vi "popElement.vi"(10 "result string 3":string, 11 "type in":i32) -> (1 "element":string, 2 "rest":string, 3 "type out":i32)   [LabVIEW 2023]
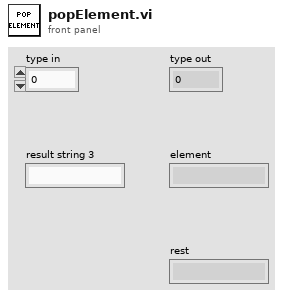
[diagram p1: front panel]
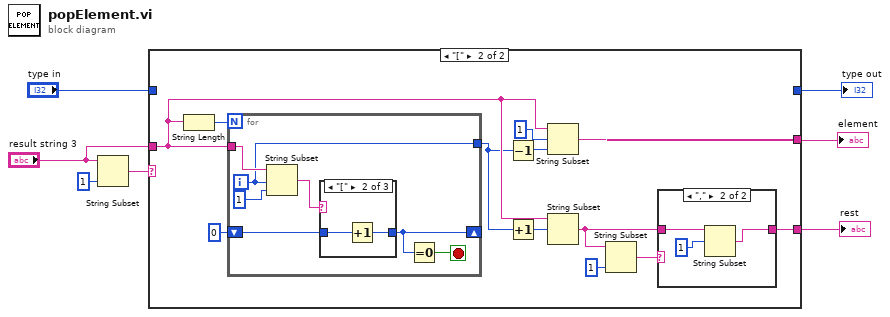
[diagram p0: block diagram]
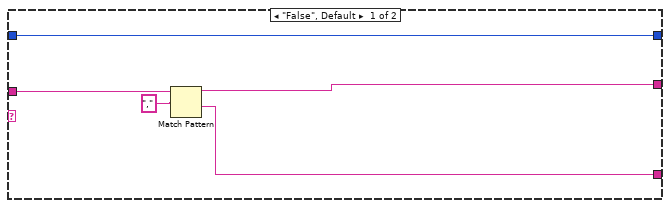
[diagram p2: hidden frame]
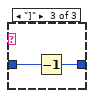
[diagram p5: hidden frame]
diagram:
  n1 = String Subset(string="result string 3", length (rest)=1 ("length (rest)")) -> (substring=w2:string)  [unwired: 1 in]
  n2 = case shown="\"[\"" w2 {
    tunnel: "result string 3" -> [w11 w21]
    tunnel: [w10 w14] -> w5
    tunnel: [w9 w20] -> w4
    tunnel: [w8 _] -> w7
    tunnel: "type in" -> [w8 _]
    frame "False", Default {
      n3 = Match Pattern(string=w11, regular expression=",") -> (before substring=w9:string, after substring=w10:string)  [unwired: 1 in, 2 out]
    }
    frame "[" {
      n4 = String Length(string=w21) -> (length=w18:i32)
      n5 = for {
        N: w18 -> [_]
        tunnel: w21 -> [w34]
        shift-right: [w31] -> _
        shift-left: 0 ("length (rest)") -> [w32]
        tunnel: [w29] -> w19
        i -> [w29]
        stop <- w30 stop-if-true
        n6 = String Subset(string=w34, offset (0)=w29, length (rest)=1 ("length (rest)")) -> (substring=w33:string)
        n7 = case shown="\"[\"" w33 {
          tunnel: w32 -> [w36 w38 w40]
          tunnel: [w36 w37 w39] -> w31
          frame "False", Default {
          }
          frame "[" {
            n8 = Increment(x=w38) -> (x+1=w37:i32)
          }
          frame "]" {
            n9 = Decrement(x=w40) -> (x-1=w39:i32)
          }
        }
        n10 = Equal To 0?(x=w31) -> (x = 0?=w30:bool)
      }
      n11 = Decrement(x=w19) -> (x-1=w22:i32)
      n12 = Increment(x=w19) -> (x+1=w17:i32)
      n13 = String Subset(string=w21, offset (0)=1, length (rest)=w22) -> (substring=w20:string)
      n14 = String Subset(string=w21, offset (0)=w17) -> (substring=w13:string)  [unwired: 1 in]
      n15 = String Subset(string=w13, length (rest)=1 ("length (rest)")) -> (substring=w15:string)  [unwired: 1 in]
      n16 = case shown="\",\"" w15 {
        tunnel: [w25 w26] -> w14
        tunnel: w13 -> [w25 w28]
        frame "not ,", Default {
        }
        frame "," {
          n17 = String Subset(string=w28, offset (0)=1) -> (substring=w26:string)  [unwired: 1 in]
        }
      }
    }
  }
  "type out" <- w7
  "rest" <- w5
  "element" <- w4
